vi "Bytes to long word.vi"(5 "Litt/BigEnd":bool, 7 "Index":i32, 9 "Image Data in":u8[](array[numeric])) -> (1 "Index+4":i32, 3 "U32":u32)   [LabVIEW 2015, in "Tiff reader.lvlib"]
doc: "Converts 4 bytes to word.\n\n\n(Inlined to prevent array extra copies)"
uses:
  Tiff reader.lvlib
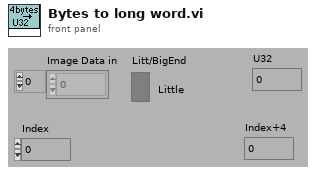
[diagram p1: front panel]
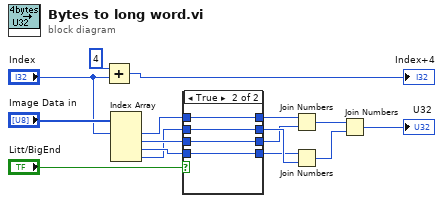
[diagram p0: block diagram]
diagram:
  n1 = Add(x=4, y="Index") -> (x+y=→"Index+4":i32)
  n2 = Index Array(array="Image Data in", index #1="Index") -> (element #1=w12:u8, element #2=w10:u8, element #3=w8:u8, element #4=w6:u8)  [unwired: 3 in]
  n3 = case shown="True" "Litt/BigEnd" {
    tunnel: w12 -> [w20 w21]
    tunnel: [w20 w24] -> w11
    tunnel: w10 -> [w19 w22]
    tunnel: [w19 w23] -> w9
    tunnel: w8 -> [w18 w23]
    tunnel: [w18 w22] -> w7
    tunnel: w6 -> [w17 w24]
    tunnel: [w17 w21] -> w5
    frame False {
    }
    frame True {
    }
  }
  n4 = Join Numbers(hi=w5, lo=w7) -> ((hi.lo)=w14:u16)
  n5 = Join Numbers(hi=w9, lo=w11) -> ((hi.lo)=w15:u16)
  n6 = Join Numbers(hi=w14, lo=w15) -> ((hi.lo)=→"U32":u32)
